vi "CompileExperimentCode.vi"(9 "ExperimentID":string, 10 "Value":string, 11 "ScriptFile":path) -> (1 "Compiled?":bool, 2 "Errors Text":string, 3 "ExperimentID":string)   [LabVIEW 2017]
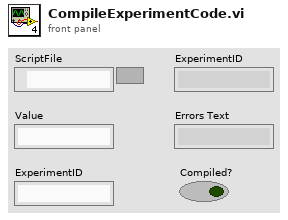
[diagram p1: front panel]
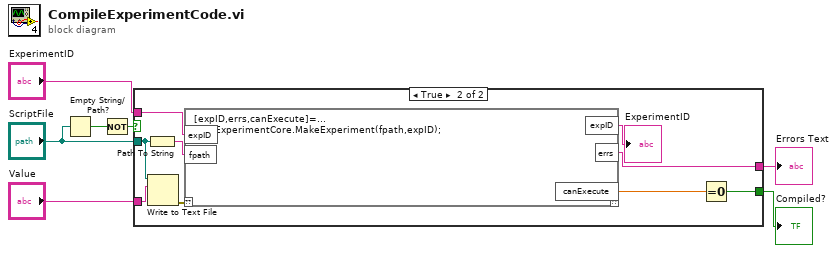
[diagram p0: block diagram]
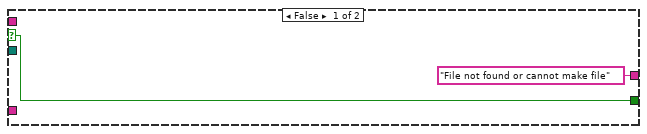
[diagram p2: hidden frame]
diagram:
  n1 = Empty String/Path?(string/path="ScriptFile") -> (empty?=w6:bool)
  n2 = Not(x=w6) -> (.not. x?=w4:bool)
  n3 = case shown="True" w4 {
    selector: w4 -> [w8 _]
    tunnel: "Value" -> [_ w18]
    tunnel: "ScriptFile" -> [_ w13]
    tunnel: "ExperimentID" -> [_ w10]
    tunnel: ["File not found or cannot make file" w17] -> w2
    tunnel: [w8 w14] -> w1
    frame False {
    }
    frame True {
      n4 = Path To String(path=w13) -> (string=w11:string)
      n5 = Write to Text File(file (use dialog)=w13, text=w18) -> (error out=w12:errorcluster)  [unwired: 2 in, 2 out]
      n6 = script code="[expID,errs,canExecute]=...\n       ExperimentCore.MakeExperiment(fpath,expID);"("??"=w12, "expID"=w10, "fpath"=w11) -> ("expID"=→"ExperimentID":string, "errs"=w17:string, "canExecute"=w15:dbl)  [unwired: 1 out]
      n7 = Equal To 0?(x=w15) -> (x = 0?=w14:bool)
    }
  }
  "Compiled?" <- w1
  "Errors Text" <- w2
